vi "Output Delay.vi"(8 "error in (no error)":errorcluster, 11 "Ramp Use Case in":refnum<class "Ramp Voltage.lvclass">) -> (0 "error out":errorcluster, 3 "Ramp Use Case out":refnum<class "Ramp Voltage.lvclass">)   [LabVIEW 2020, in "High Level PSU With Tests.lvlib" / "Ramp Voltage.lvclass"]
uses:
  Ramp Voltage.lvclass
  Ramp Voltage.lvclass/Ramp Voltage.ctl
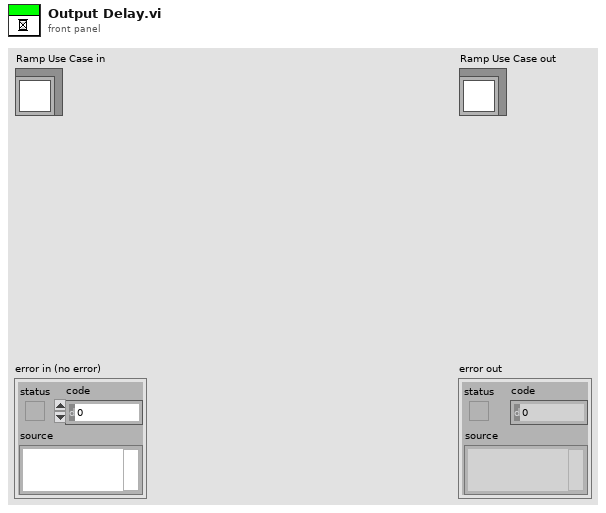
[diagram p1: front panel]
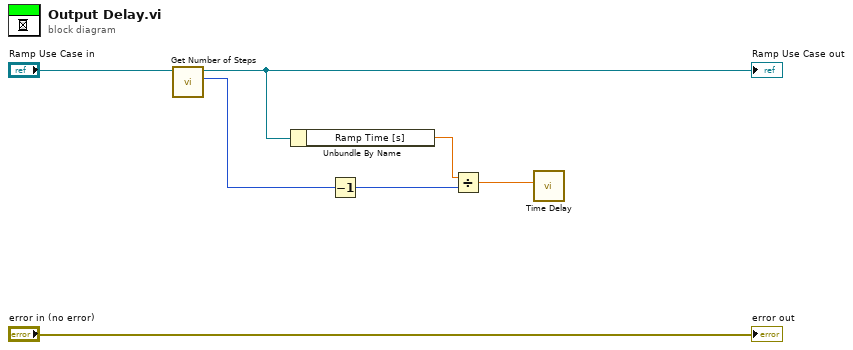
[diagram p0: block diagram]
diagram:
  n1 = call "Get Number of Steps.vi"("Ramp Use Case in"="Ramp Use Case in") -> ("Numeric"=w3:i32, "Ramp Use Case out"=w5:refnum<class "Ramp Voltage.lvclass">)  [unwired: 8 in, 1 out]
  "Ramp Use Case out" <- w5
  n2 = Unbundle By Name(w5) -> ("Ramp Time [s]"=w4:dbl)
  n3 = Decrement(x=w3) -> (x-1=w2:i32)
  n4 = Divide(x=w4, y=w2) -> (x/y=w1:dbl)
  n5 = call "Time Delay"("Delay Time (s)"=w1) -> ()  [unwired: 10 in, 1 out]
  "error out" <- "error in (no error)"
